vi "uintArraySort.vi"(8 "Error in (no error)":errorcluster, 11 "Uint array in":refnum<class "UintClass.lvclass">[](array[class])) -> (0 "Error out":errorcluster, 1 "Timing":u32, 3 "Sorted uint array":refnum<class "UintClass.lvclass">[](array[class]))   [LabVIEW 2011, in "UintClass.lvclass"]
uses:
  UintClass.lvclass
  uintGreater.vi
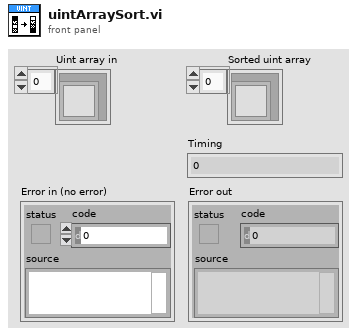
[diagram p1: front panel]
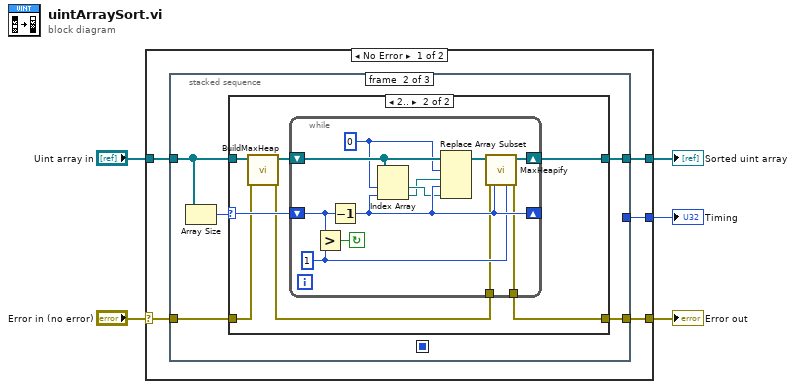
[diagram p0: block diagram]
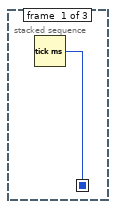
[diagram p2: hidden frame]
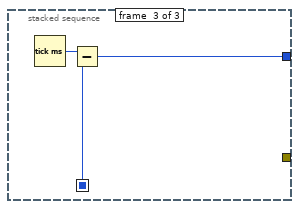
[diagram p4: hidden frame]
diagram:
  n1 = case shown="No Error" "Error in (no error)" {
    selector: "Error in (no error)" -> [w8 w41]
    tunnel: "Uint array in" -> [w10 _]
    tunnel: [w9 _] -> w3
    tunnel: [w7 w41] -> w2
    tunnel: [w6 _] -> w1
    frame No Error {
      n2 = stacked-sequence {
        seq-local: [w11 _ _] -> [_ _ w39]
        tunnel: w10 -> [_ w15 _]
        tunnel: [_ w14 _] -> w9
        tunnel: w8 -> [_ w13 _]
        tunnel: [_ w12 _] -> w7
        tunnel: [_ _ w38] -> w6
        frame #0 {
          n3 = Tick Count (ms)() -> (millisecond timer value=w11:u32)
        }
        frame #1 {
          n4 = Array Size(array=w15) -> (size(s)=w16:i32)
          n5 = case shown="2.." w16 {
            selector: w16 -> [_ w22]
            tunnel: [w18 w24] -> w14
            tunnel: w15 -> [w18 w23]
            tunnel: w13 -> [w17 w21]
            tunnel: [w17 w19] -> w12
            frame ..1 {
            }
            frame 2.. {
              n6 = call "BuildMaxHeap.vi"("Error in (no error)"=w21, "Heap in"=w23) -> ("Error out"=w20:errorcluster, "Heap out"=w25:refnum<class "UintClass.lvclass">[])  [unwired: 8 in]
              n7 = while {
                shift-right: [w31] -> _
                shift-left: w22 -> [w36]
                shift-right: [w34] -> w24
                shift-left: w25 -> [w33]
                tunnel: w20 -> [w27]
                tunnel: [w26] -> w19
                stop <- w37 continue-if-true
                w32 = 0 ("index")
                w28 = 1 ("y")
                n8 = Greater?(x=w36, y=w28) -> (0:w37:bool)
                n9 = Decrement(x=w36) -> (x-1=w31:i32)
                n10 = Index Array(array=w33, index #1=w32, index #2=w31) -> (element #1=w30:refnum<class "UintClass.lvclass">, element #2=w29:refnum<class "UintClass.lvclass">)
                n11 = Replace Array Subset(array=w33, new element #1=w29, index #1=w32, new element #2=w30, index #2=w31) -> (w35:refnum<class "UintClass.lvclass">[])
                n12 = call "MaxHeapify.vi"("Error in (no error)"=w27, "Length"=w31, "i"=w28, "Heap in"=w35) -> ("Error out"=w26:errorcluster, "Heap out"=w34:refnum<class "UintClass.lvclass">[])  [unwired: 6 in]
              }
            }
          }
        }
        frame #2 {
          n13 = Tick Count (ms)() -> (millisecond timer value=w40:u32)
          n14 = Subtract(x=w40, y=w39) -> (x-y=w38:u32)
        }
      }
    }
    frame Error {
    }
  }
  "Sorted uint array" <- w3
  "Error out" <- w2
  "Timing" <- w1
